vi "AH_GetGlobals.vi"(8 "error in (no error)":errorcluster, 9 "Data_In":T1 {"GUI Data Cluster"."SBR" format="%08b"}, 10 "Cluster IN":T3={"General"={"Config.ini"=path "", "Default Logging Path"=path ""}, "Hardware"={"AHC VISA COM"="", "Measure Rate (1/s)"=0, "Global T VAR"="", "Global B VAR"="", "Average"=4, "Bias"=0, "Cable"={"Length"=0.0, "Resistance"=0.0, "Inductance"=0.0, "Capacitance"=0.0}, "Tracking"=0, "Voltage"=0.0}, "Operation"={"Operation Mode"=enum."Idle-Off", "Status"="", "NewLog?"=FALSE, "OvenWarn"=FALSE}}, 11 "Start Stamp":timestamp) -> (0 "error out":errorcluster, 1 "Data_Out":T1 {"GUI Data Cluster"."SBR" format="%08b"}, 2 "Cluster OUT":T3={"General"={"Config.ini"=path "", "Default Logging Path"=path ""}, "Hardware"={"AHC VISA COM"="", "Measure Rate (1/s)"=0, "Global T VAR"="", "Global B VAR"="", "Average"=4, "Bias"=0, "Cable"={"Length"=0.0, "Resistance"=0.0, "Inductance"=0.0, "Capacitance"=0.0}, "Tracking"=0, "Voltage"=0.0}, "Operation"={"Operation Mode"=enum."Idle-Off", "Status"="", "NewLog?"=FALSE, "OvenWarn"=FALSE}}, 4 "T Var":dbl, 5 "T Delta t":dbl, 6 "B Var":dbl, 7 "B Delta t":dbl)   [LabVIEW 2021]
uses:
  Config_Cluster.ctl
  Mode_Enum.ctl
  Data_Cluster.ctl
  Measurement_Cluster.ctl
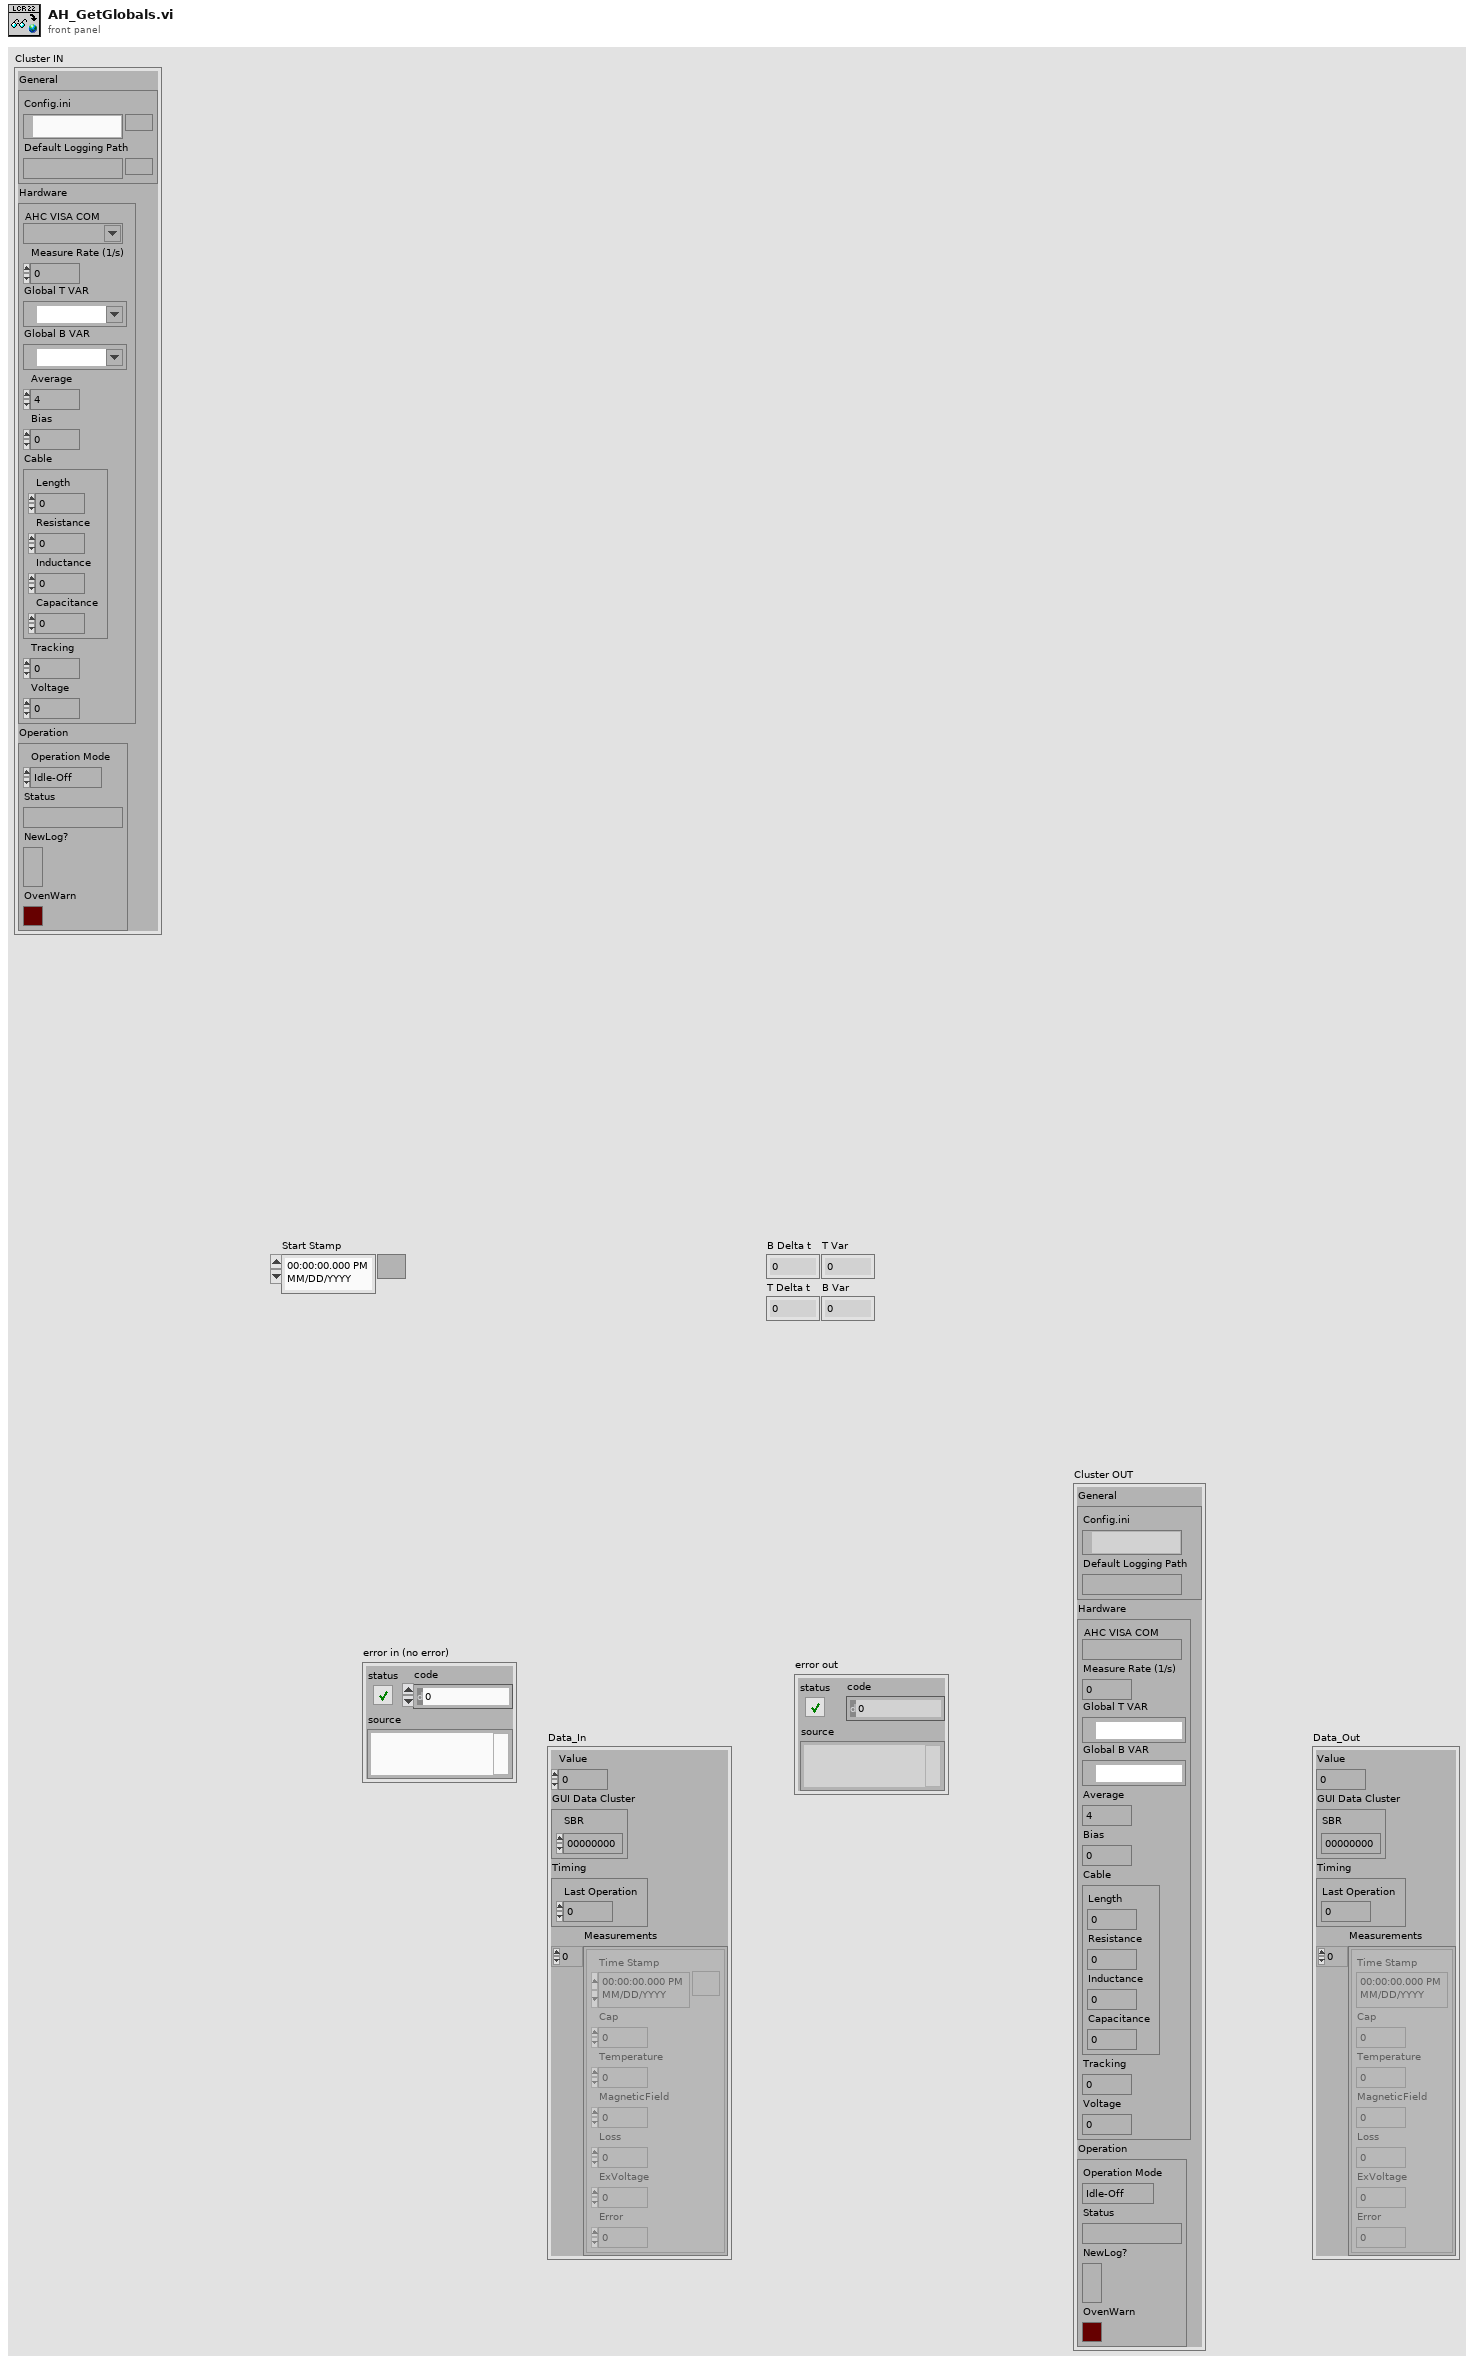
[diagram p1: front panel]
types:
  T1 = typedef "Data_Cluster.ctl" = cluster{"Value":dbl, "GUI Data Cluster":cluster{"SBR":u16}, "Timing":cluster{"Last Operation":dbl}, "Measurements":T2[]}
  T2 = typedef "Measurement_Cluster.ctl" = cluster{"Time Stamp":timestamp, "Cap":dbl, "Temperature":dbl, "MagneticField":dbl, "Loss":dbl, "ExVoltage":dbl, "Error":dbl}
  T3 = typedef "Config_Cluster.ctl" = cluster{"General":cluster{"Config.ini":path, "Default Logging Path":path}, "Hardware":cluster{"AHC VISA COM":refnum<visa-resource-name>, "Measure Rate (1/s)":i32, "Global T VAR":refnum<k21>, "Global B VAR":refnum<k21>, "Average":u8, "Bias":u8, "Cable":cluster{"Length":dbl, "Resistance":dbl, "Inductance":dbl, "Capacitance":dbl}, "Tracking":u8, "Voltage":dbl}, "Operation":cluster{"Operation Mode":T4, "Status":string, "NewLog?":bool, "OvenWarn":bool}}
  T4 = typedef "Mode_Enum.ctl" = enum16{"OvenNRDY", "Logging", "Idle-Off", "Idle"}
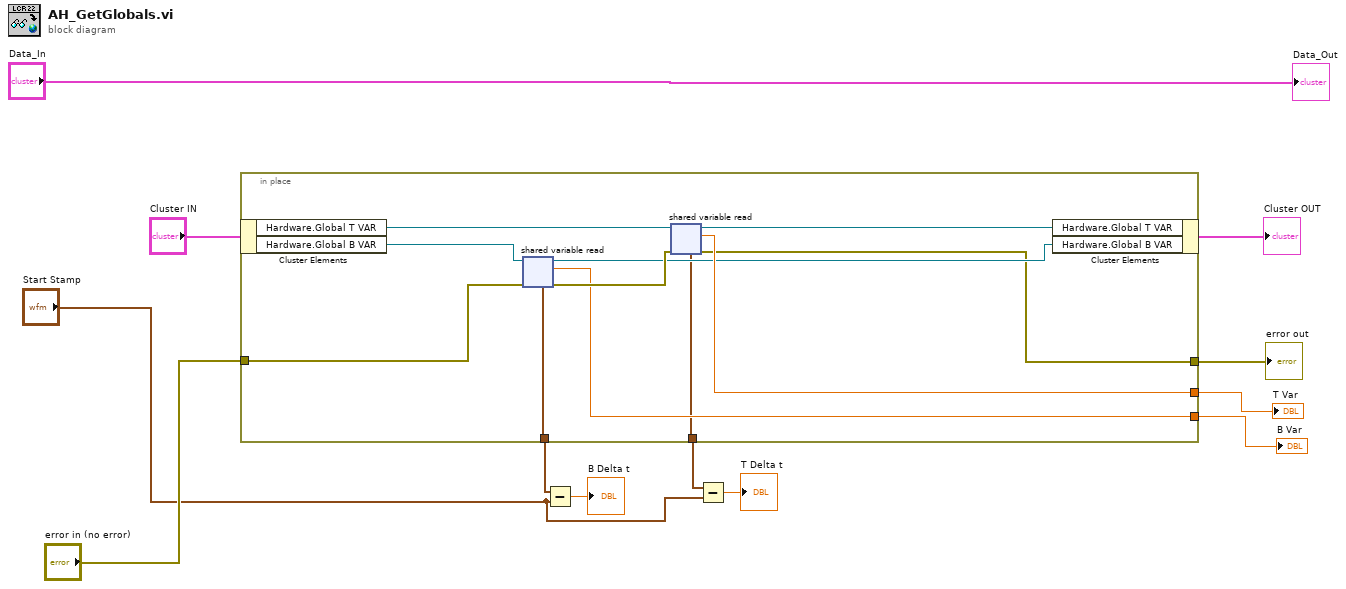
[diagram p0: block diagram]
diagram:
  n1 = in-place {
    in-place-border: "error in (no error)" -> [w22]
    in-place-border: [w19] -> w1
    in-place-border: [w18] -> w2
    in-place-border: [w15] -> w8
    in-place-border: [w14] -> w7
    in-place-border: [w13] -> w5
    n2 = in-place-cluster #1("Cluster IN") -> ("Hardware.Global T VAR"=w21:refnum<k21>, "Hardware.Global B VAR"=w23:refnum<k21>)
    n3 = shared-variable-read(w23, w22) -> (w16:refnum<k21>, w20:errorcluster, w19:dbl, w14:timestamp)
    n4 = shared-variable-read(w21, w20) -> (w17:refnum<k21>, w15:errorcluster, w18:dbl, w13:timestamp)
    n5 = in-place-cluster #1("Hardware.Global T VAR"=w17, "Hardware.Global B VAR"=w16) -> (→"Cluster OUT":T3)
  }
  "error out" <- w8
  "T Var" <- w2
  "B Var" <- w1
  n6 = Subtract(x=w7, y="Start Stamp") -> (x-y=→"B Delta t":dbl)
  n7 = Subtract(x=w5, y="Start Stamp") -> (x-y=→"T Delta t":dbl)
  "Data_Out" <- "Data_In"
